vi "KB-计算象限最大值.vi"(8 "个数":i32, 9 "列":i32, 10 "行":i32, 11 "內圆数组":dbl[][](array[numeric])) -> (3 "象限最大值":dbl)   [LabVIEW 2015]
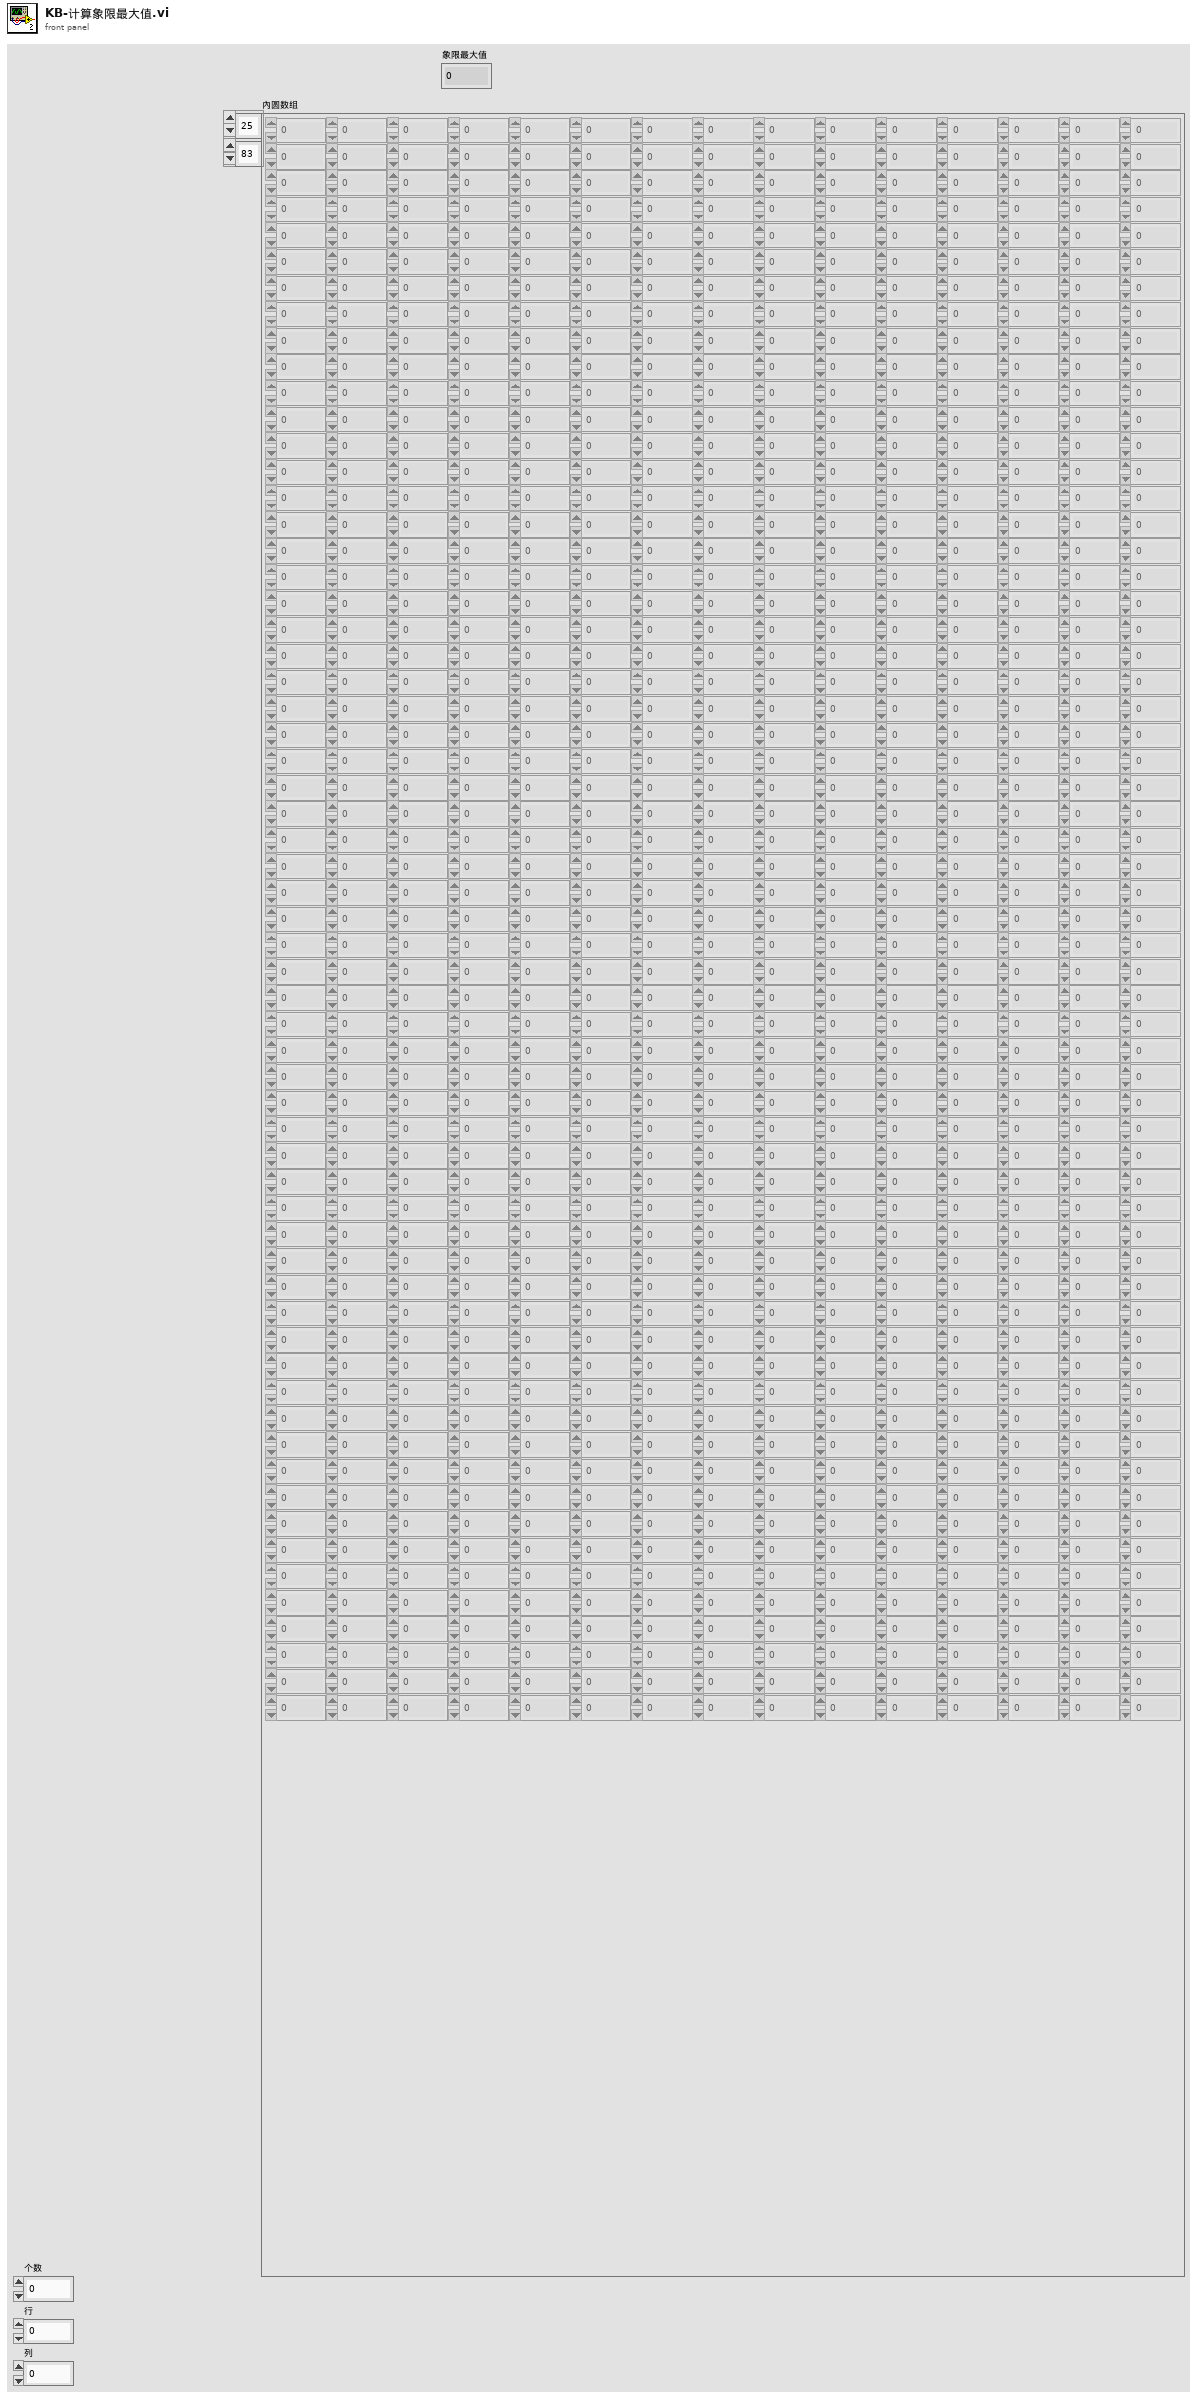
[diagram p1: front panel]
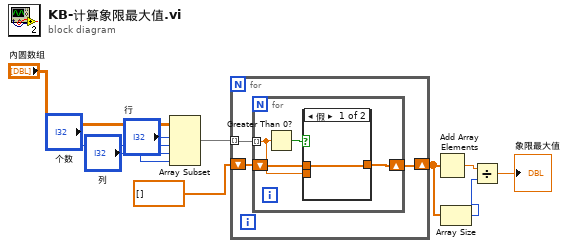
[diagram p0: block diagram]
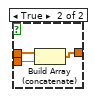
[diagram p2: hidden frame]
diagram:
  n1 = Array Subset(array="內圆数组", index (row)="行", length (row)="个数", index (col)="列", length (col)="个数") -> (w10:dbl[][])
  n2 = for {
    tunnel: w10 -> [w13] mode=indexing
    shift-right: [w11] -> w8
    shift-left: dbl[] [] -> [w12]
    n3 = for {
      tunnel: w13 -> [w14] mode=indexing
      shift-right: [w15] -> w11
      shift-left: w12 -> [w17]
      n4 = Greater Than 0?(x=w14) -> (x > 0?=w16:bool)
      n5 = case shown="假" w16 {
        tunnel: w17 -> [w18 w21]
        tunnel: [w18 w20] -> w15
        tunnel: w14 -> [_ w19]
        frame False {
        }
        frame True {
          n6 = Build Array (concatenate)(w21, w19) -> (w20:dbl[])
        }
      }
    }
  }
  n7 = Add Array Elements(numeric array=w8) -> (sum=w7:dbl)
  n8 = Array Size(array=w8) -> (size(s)=w6:i32)
  n9 = Divide(x=w7, y=w6) -> (x/y=→"象限最大值":dbl)
